vi "FTW-ScheduledJob-ReadyOrNot.vi"(0 "FTW Scheduled Job":refnum<class "FTW-ScheduledJob.lvclass">, 11 "error in":errorcluster) -> (4 "FTW Scheduled Job out":refnum<class "FTW-ScheduledJob.lvclass">, 6 "Next Schedule Deadline":u32 format="%d msec", 8 "Next Schedule Active":bool, 10 "Ready to Schedule":bool, 15 "error out":errorcluster)   [LabVIEW 2015, in "FTW-ScheduledJob.lvclass"]
uses:
  FTW-ScheduledJob.lvclass
panel:
  # "Inputs"
  # "Outputs"
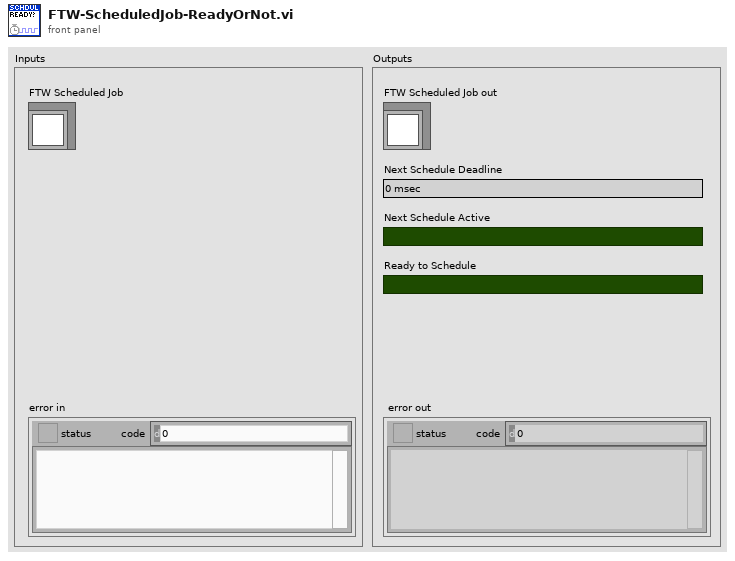
[diagram p1: front panel]
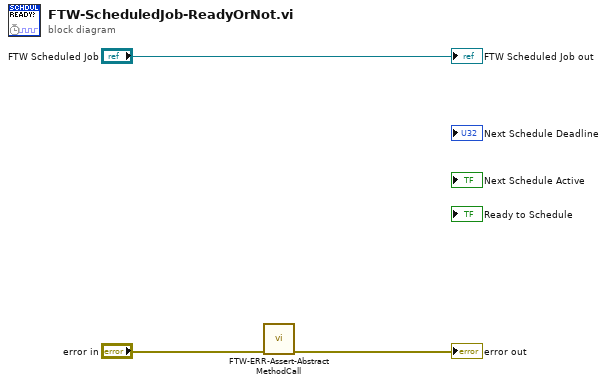
[diagram p0: block diagram]
diagram:
  n1 = call "FTW-ERR-Assert-AbstractMethodCall.vi"("error in"="error in") -> ("error out"=→"error out":errorcluster)  [unwired: 14 in]
  "FTW Scheduled Job out" <- "FTW Scheduled Job"
